vi "SubVI Tester.vi"() -> ()   [LabVIEW 2022 SP3]
uses:
  Weather Data.ctl
panel:
  out "Weather Data Out":T1={"Current Temperature"=0.0, "Max Temperature"=0.0, "Min Temperature"=0.0, "Temperature Warning?"=FALSE, "Temperature Warning Text"="No Warning", "Units"=enum."Celsius"}
  in  "Min Temperature":dbl=10.0
  in  "Max Temperature":dbl=30.0
  in  "Stop":bool
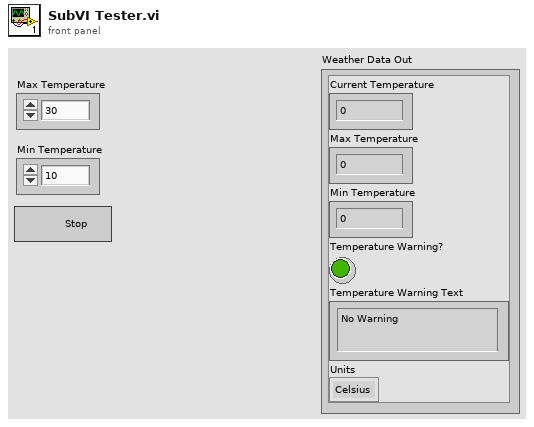
[diagram p1: front panel]
types:
  T1 = typedef "Weather Data.ctl" = cluster{"Current Temperature":dbl, "Max Temperature":dbl, "Min Temperature":dbl, "Temperature Warning?":bool, "Temperature Warning Text":string, "Units":enum16{"Celsius", "Fahrenheit"}}
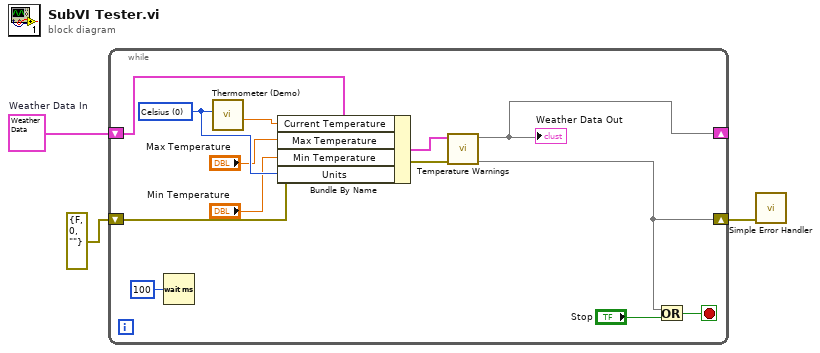
[diagram p0: block diagram]
diagram:
  w1 = T1 {"Current Temperature"=20.0, "Max Temperature"=18.0, "Min Temperature"=10.0, "Temperature Warning?"=FALSE, "Temperature Warning Text"="No Warning", "Units"=enum."Celsius"}  # Weather Data In
  n1 = while {
    shift-right: [w4] -> w3
    shift-left: errorcluster {"status"=FALSE, "code"=0, "source"=""} ("error in") -> [w6]
    shift-right: [w5] -> _
    shift-left: w1 -> [w12]
    stop <- w13 stop-if-true
    w11 = u16 0 items=["Celsius", "Fahrenheit"] ("Units (0: Celsius)")
    n2 = Wait (ms)(milliseconds to wait=u32 100) -> ()  [unwired: 1 out]
    n3 = call "Thermometer (Demo).vi"("Units (0: Celsius)"=w11) -> ("Temperature Value"=w8:dbl)  [unwired: 10 in]
    n4 = Bundle By Name(cluster=w12, "Current Temperature"=w8, "Max Temperature"="Max Temperature", "Min Temperature"="Min Temperature", "Units"=w11) -> (w7:T1)
    n5 = call "Temperature Warnings.vi"(8:w6, 11:w7) -> (0:w4, 3:w5)  [unwired: 8 in]
    "Weather Data Out" <- w5
    n6 = Or(x=w4, y="Stop") -> (x .or. y?=w13:bool)
  }
  n7 = call <vilib>:"Simple Error Handler.vi"("error in (no error)"=w3) -> ()  [unwired: 4 in, 5 out]
